vi "Send Host Stream Command Exit.vi"(8 "error in (no error)":errorcluster, 11 "Q Refs":T1) -> (0 "error out":errorcluster)   [LabVIEW 2019, in "CAN Stream Support Workspace Shared.lvlib"]
uses:
  CAN Stream Support Workspace Shared.lvlib
  Types/Host Stream Queue Refs.ctl
  Types/Host Stream Queue Type.ctl
  Types/Host Stream Queue Command.ctl
  <vilib>/xnet/xnet.llb/XNET Frame CAN.ctl
  <vilib>/xnet/xnet.llb/XNET Frame Type CAN.ctl
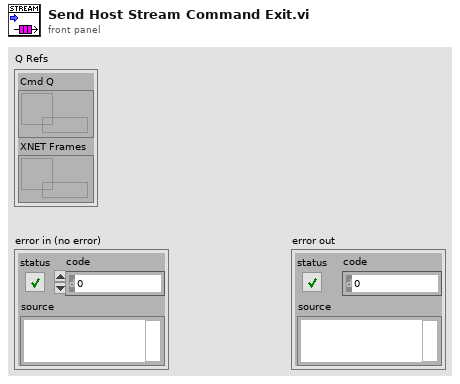
[diagram p1: front panel]
types:
  T1 = typedef "CAN Stream Support Workspace Shared.lvlib/Host Stream Queue Refs.ctl" = cluster{"Cmd Q":refnum<queue>, "XNET Frames":refnum<queue>}
  T2 = typedef "CAN Stream Support Workspace Shared.lvlib/Host Stream Queue Type.ctl" = cluster{"Cmd":T3, "Target IP Address":string, "Addon":string}
  T3 = typedef "CAN Stream Support Workspace Shared.lvlib/Host Stream Queue Command.ctl" = enum8{"Start Stream", "Stop Stream", "Exit"}
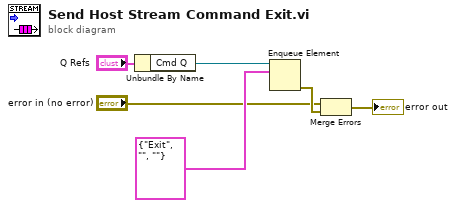
[diagram p0: block diagram]
diagram:
  n1 = Unbundle By Name("Q Refs") -> ("Cmd Q"=w1:refnum<queue>)
  n2 = Enqueue Element(queue=w1, element=T2 {"Cmd"=enum."Exit", "Target IP Address"="", "Addon"=""}) -> (error out=w4:errorcluster)  [unwired: 2 in, 2 out]
  n3 = Merge Errors("error in (no error)", w4) -> (→"error out":errorcluster)
